vi "FGV_PSP - Mercury Action Status.vi"(4 "error in":errorcluster, 6 "Function":enum16{"write", "read"}(ring), 7 "Mercury Status":string) -> (0 "error out":errorcluster, 3 "Mercury Status 2":string)   [LabVIEW 2013]
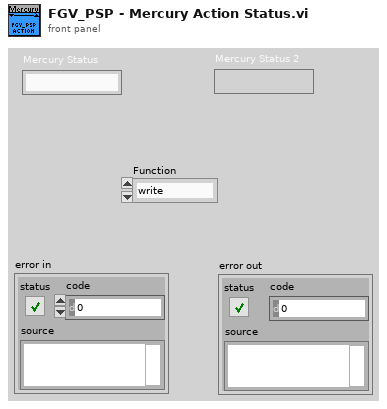
[diagram p1: front panel]
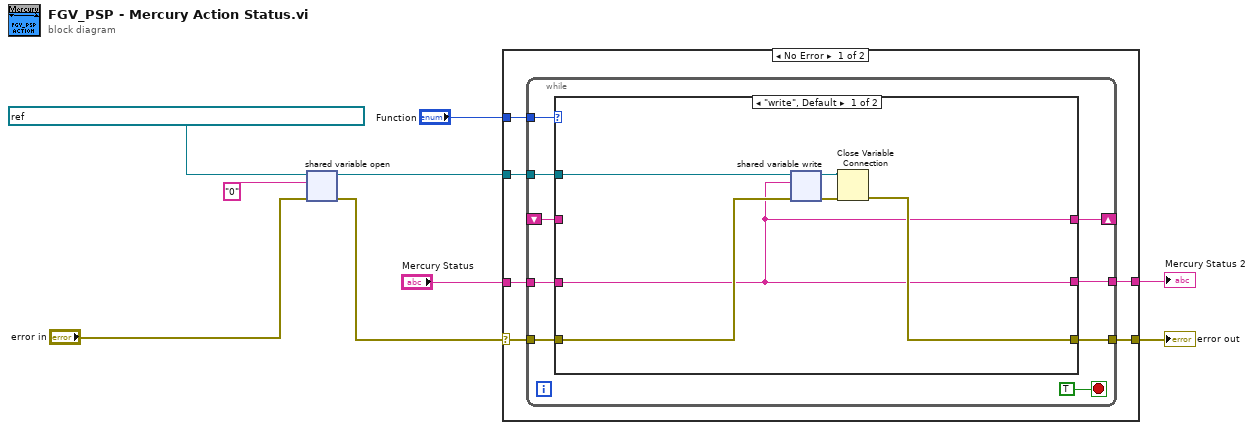
[diagram p0: block diagram]
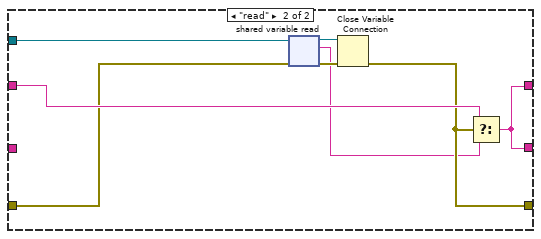
[diagram p2: hidden frame]
diagram:
  n1 = shared-variable-open(refnum<k21> "ni.var.psp://localhost/1820/Mercury_Status" ("shared variable refnum in"), "error in", "0" ("Mercury Status")) -> (w7:refnum<k21>, w3:errorcluster)  [unwired: 1 in]
  n2 = case shown="No Error" w3 {
    selector: w3 -> [w15 w40]
    tunnel: [w14 w40] -> w9
    tunnel: [w13 w39] -> w6
    tunnel: "Function" -> [w12 _]
    tunnel: w7 -> [w11 _]
    tunnel: "Mercury Status" -> [w10 w39]
    frame No Error {
      n3 = while {
        shift-right: [w19] -> _
        shift-left: _ -> [w18]
        tunnel: w15 -> [w23]
        tunnel: [w22] -> w14
        tunnel: [w21] -> w13
        tunnel: w12 -> [w20]
        tunnel: w11 -> [w17]
        tunnel: w10 -> [w16]
        stop <- TRUE stop-if-true
        n4 = case shown="\"write\", Default" w20 {
          tunnel: w23 -> [w27 w32]
          tunnel: [w29 w34] -> w22
          tunnel: [w25 w35] -> w21
          tunnel: [w25 w35] -> w19
          tunnel: w18 -> [_ w36]
          tunnel: w17 -> [w26 w33]
          tunnel: w16 -> [w25 _]
          frame "write", Default {
            n5 = shared-variable-write(w26, w27, w25) -> (w28:refnum<k21>, w30:errorcluster)
            n6 = Close Variable Connection(8:w30, 11:w28) -> (0:w29:errorcluster)
          }
          frame "read" {
            n7 = shared-variable-read(w33, w32) -> (w38:refnum<k21>, w37:errorcluster, w31:string)  [unwired: 1 out]
            n8 = Close Variable Connection(8:w37, 11:w38) -> (0:w34:errorcluster)
            n9 = Select(t=w36, s=w34, f=w31) -> (s? t:f=w35:string)
          }
        }
      }
    }
    frame Error {
    }
  }
  "error out" <- w9
  "Mercury Status 2" <- w6
